vi "P3060_根据资源名称打开设备.vi"(8 "error in (no error)":errorcluster caption="错误输入（无错误）", 11 "设备资源名称":string) -> (0 "error out":errorcluster caption="错误输出", 3 "句柄输出":i32)   [LabVIEW 2010]
doc: "根据设备资源名称打开板卡！"
uses:
  _SubVI/dll/P3060.dll
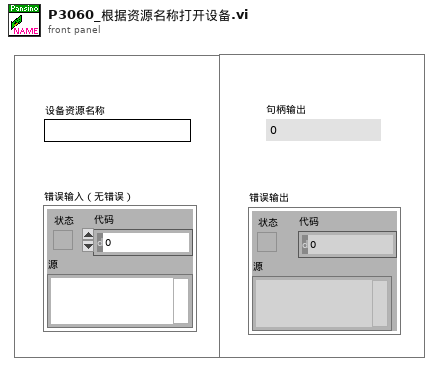
[diagram p1: front panel]
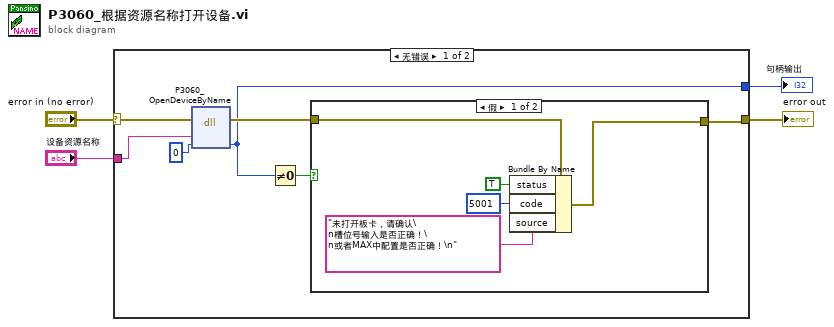
[diagram p0: block diagram]
diagram:
  n1 = case shown="无错误" "error in (no error)" {
    selector: "error in (no error)" -> [w11 w18]
    tunnel: [w8 w18] -> w3
    tunnel: [w7 _] -> w2
    tunnel: "设备资源名称" -> [w5 _]
    frame No Error {
      n2 = dll-call lib="D:/driver/trunk/Drivers/P3060/P3060API/P3060APILV/Labview/P3060/_SubVI/dll/P3060.dll" fn="P3060_OpenDeviceByName"(error in=w11, "资源名称"=w5, "设备句柄"=0) -> (error out=w9:errorcluster, "设备句柄"=w7:i32)  [unwired: 4 in, 1 out]
      n3 = Not Equal To 0?(x=w7) -> (x != 0?=w10:bool)
      n4 = case shown="假" w10 {
        tunnel: w9 -> [w16 w17]
        tunnel: [w12 w17] -> w8
        frame False {
          n5 = Bundle By Name(cluster=w16, "status"=TRUE, "code"=5001, "source"="未打开板卡，请确认\n槽位号输入是否正确！\n或者MAX中配置是否正确！\n") -> (w12:errorcluster)
        }
        frame True {
        }
      }
    }
    frame Error {
    }
  }
  "error out" <- w3
  "句柄输出" <- w2
